vi "SetClassQueue.vi"(8 "ErrorIn(No Error)":errorcluster caption="entrée d'erreur (pas d'erreur)", 11 "EGG5210.lvclass":refnum<class "EGG5210.lvclass">) -> (0 "sortie d'erreur":errorcluster, 3 "EGG5210.lvclass Out":refnum<class "EGG5210.lvclass">)   [LabVIEW 2012, in "EGG5210.lvclass"]
uses:
  EGG5210.lvclass
  BaseDevice/BaseDevice.lvclass
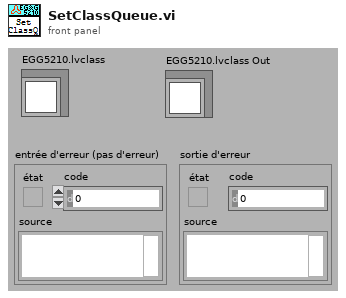
[diagram p1: front panel]
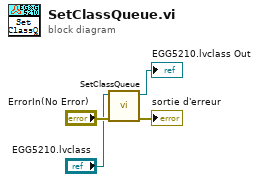
[diagram p0: block diagram]
diagram:
  n1 = call-parent "SetClassQueue.vi"("ErrorIn(No Error)"="ErrorIn(No Error)", "BaseDevice.lvclass"="EGG5210.lvclass") -> ("sortie d'erreur"=→"sortie d'erreur":errorcluster, "BaseDevice.lvclass Out"=→"EGG5210.lvclass Out":refnum<class "EGG5210.lvclass">)  [unwired: 8 in]
